vi "Get Status.vi"(8 "error in":errorcluster) -> (0 "error out":errorcluster, 3 "Messages":i32)   [LabVIEW 2025, in "Automotive Ethernet Bus Monitor.lvclass"]
doc: "Get the number of frames in the buffer queue."
uses:
  Automotive Ethernet Bus Monitor.lvclass
  Automotive Ethernet Bus Monitor.lvclass/Automotive Ethernet Bus Monitor.ctl
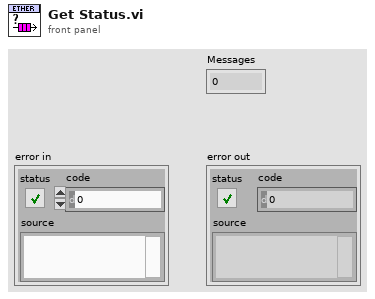
[diagram p1: front panel]
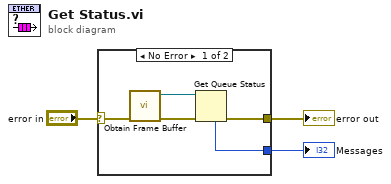
[diagram p0: block diagram]
diagram:
  n1 = case shown="No Error" "error in" {
    selector: "error in" -> [w8 w9]
    tunnel: [w5 w9] -> w2
    tunnel: [w4 _] -> w1
    frame No Error {
      n2 = call "Obtain Frame Buffer.vi"("error in"=w8) -> ("error out"=w6:errorcluster, "queue out"=w7:refnum<queue>)  [unwired: 9 in]
      n3 = Get Queue Status(queue=w7, error in (no error)=w6) -> (error out=w5:errorcluster, # elements in queue=w4:i32)  [unwired: 1 in, 6 out]
    }
    frame Error {
    }
  }
  "error out" <- w2
  "Messages" <- w1
